vi "Fetch Multi Eval Meas List Segment Power Monitor RMS Results.vi"(8 "error in (no error)":errorcluster, 9 "Segment (1)":T2=1, 10 "Instance (1)":T3=1, 11 "VISA resource name":refnum<visa-resource-name>) -> (0 "error out":errorcluster, 1 "Results":dbl[](array[numeric]) format="%^.3e", 2 "Reliability":T1, 3 "VISA resource name out":refnum<visa-resource-name>)   [LabVIEW 2020, in "Rohde&Schwarz CMWXP NR FR1 Measurement.lvlib"]
doc: "Return the power monitor results for segment <no> in list mode. The commands return one power result for each subframe of the segment for the measured carrier. The power values are RMS averaged over the subframe.\n\nAttribute:\nRSCMWXPNRFR1M_ATTR_FETCH_MULTI_EVAL_MEAS_LIST_SEGMENT_POWER_MONITOR_RMS_RESULTS\n\nRemote-control command:\nFETCh:NRSub:MEAS<i>:MEValuation:LIST:SEGMent<no>:PMONitor:RMS?"
uses:
  <instrlib>/Rohde&Schwarz CMWXP NR FR1 Measurement/Rohde&Schwarz CMWXP NR FR1 Measurement.lvlib
  <instrlib>/Rohde&Schwarz CMWXP NR FR1 Measurement/Private/_Instance.ctl
  <instrlib>/Rohde&Schwarz CMWXP NR FR1 Measurement/Private/_Segment.ctl
  <instrlib>/Rohde&Schwarz CMWXP NR FR1 Measurement/Private/_SegReliability.ctl
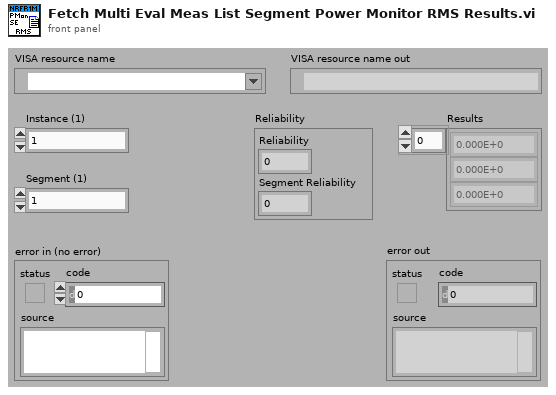
[diagram p1: front panel]
types:
  T1 = typedef "Rohde&Schwarz CMWXP NR FR1 Measurement.lvlib/_SegReliability.ctl" = cluster{"Reliability":i32, "Segment Reliability":i32}
  T2 = typedef "Rohde&Schwarz CMWXP NR FR1 Measurement.lvlib/_Segment.ctl" = i32
  T3 = typedef "Rohde&Schwarz CMWXP NR FR1 Measurement.lvlib/_Instance.ctl" = i32
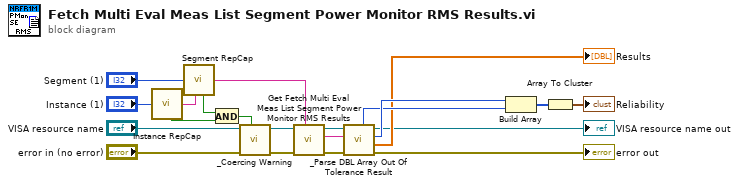
[diagram p0: block diagram]
diagram:
  n1 = call <instrlib>:"Instance RepCap.vi"("Instance In"="Instance (1)") -> ("In Range?"=w16:bool, "RepCap Identifier Out"=w15:string)  [unwired: 1 in]
  n2 = call <instrlib>:"Segment RepCap.vi"("Segment In"="Segment (1)", "RepCap String In (\"\")"=w15) -> ("In Range?"=w14:bool, "RepCap Identifier Out"=w13:string)
  n3 = And(x=w14, y=w16) -> (x .and. y?=w17:bool)
  n4 = call <instrlib>:"_Coercing Warning.vi"("In Range?"=w17, "error in (no error)"="error in (no error)", "VISA resource name"="VISA resource name") -> ("error out"=w11:errorcluster, "VISA resource name out"=w12:refnum<visa-resource-name>)  [unwired: 7 in]
  n5 = call "Get Fetch Multi Eval Meas List Segment Power Monitor RMS Results"("Repeated Capabilities"=w13, "error in (no error)"=w11, "instrument handle"=w12) -> ("error out"=w8:errorcluster, "Fetch Multi Eval Meas List Segment Power Monitor RMS Results"=w9:string, "instrument handle out"=w10:refnum<visa-resource-name>)  [unwired: 6 in]
  n6 = call <instrlib>:"_Parse DBL Array Out Of Tolerance Result.vi"("error in (no error)"=w8, "Input String"=w9, "VISA resource name"=w10) -> ("error out"=→"error out":errorcluster, "Results"=→"Results":dbl[], "Reliability"=w5:i32, "VISA resource name out"=→"VISA resource name out":refnum<visa-resource-name>, "Out Of Tolerance"=w4:i32)  [unwired: 4 in]
  n7 = Build Array(w5, w4) -> (w6:i32[])
  n8 = Array To Cluster(array=w6) -> (cluster=→"Reliability":cluster{"[0]":i32, "[1]":i32})
